vi "Read Osc Waveform.vi"(0 "RedPitaya TCP Connection in":refnum<k5>, 5 "error in":errorcluster, 6 "Channel #":u16(ring) items=["Channel 1", "Channel 2"], 12 "timeout ms (2000)":i32) -> (14 "RedPitaya TCP Connection out":refnum<k5>, 16 "Measurement Array":sgl[](array[numeric]), 19 "error out":errorcluster)   [LabVIEW 8.6]
doc: "Read the data stream of the data currently “displayed”."
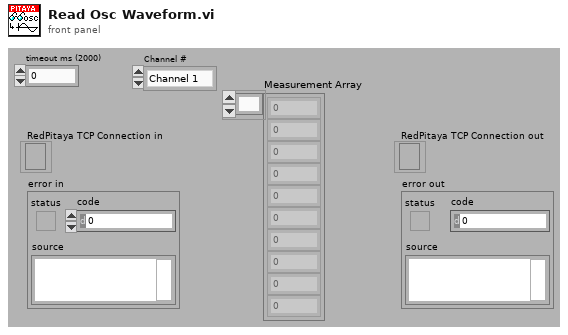
[diagram p1: front panel]
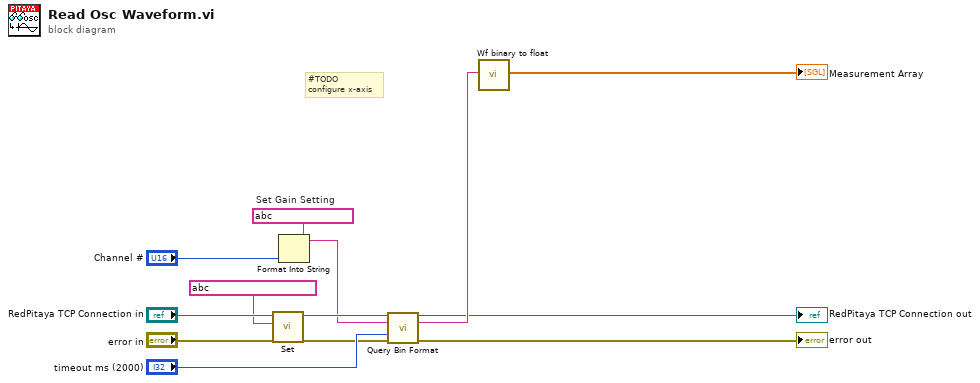
[diagram p0: block diagram]
diagram:
  w13 = string ?  # Set Gain Setting
  # "#TODO\nconfigure x-axis"
  n1 = call "Set.vi"("error in"="error in", "SCPI Message"=string ?, "RedPitaya connection in"="RedPitaya TCP Connection in") -> ("error out"=w5:errorcluster, "RedPitaya connection out"=w8:refnum<k5>)  [unwired: 6 in, 1 out]
  n2 = Format Into String(format string=w13, "Channel #") -> (resulting string=w7:string)  [unwired: 2 in, 1 out]
  n3 = call "Query Bin Format.vi"("RedPitaya connection in"=w8, "SCPI Query"=w7, "timeout ms (2000)"="timeout ms (2000)", "error in"=w5) -> ("RedPitaya connection out"=→"RedPitaya TCP Connection out":refnum<k5>, "data out"=w4:string, "error out"=→"error out":errorcluster)  [unwired: 9 in]
  n4 = call "Wf binary to float.vi"("Input string"=w4) -> ("Data out"=→"Measurement Array":sgl[])  [unwired: 18 in]
